vi "Stop Core.vi"(10 "final error code":i32, 11 "CS++RTRootActor in":refnum<class "CS++RTRootActor.lvclass">) -> (3 "CS++RTRootActor out":refnum<class "CS++RTRootActor.lvclass">)   [LabVIEW 2014, in "CS++RTRoot.lvlib" / "CS++RTRootActor.lvclass"]
doc: "(<B>Filename</B>: Actor Framework.lvlib:Actor.lvclass:Stop Core.vi)\n\nDefines what the actor does before it stops. Use the <B>final error code</B> input to determine whether the actor shut down in response to an error.\n\nBy default, this method does nothing. A descendant class may override it to define behavior, such as shutting down any processes the actor initiated in its override of the Actor Core method."
uses:
  CS++RTRootActor.lvclass
  <vilib>/ActorFramework/Actor/Actor.lvclass
  CSPP_Core/Libraries/Utilities/CS++Utilities.lvlib
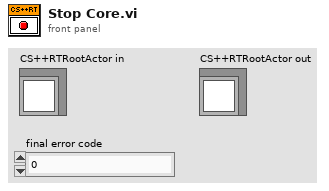
[diagram p1: front panel]
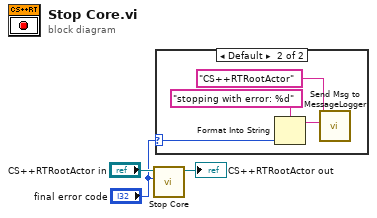
[diagram p0: block diagram]
diagram:
  n1 = call-parent "Stop Core.vi"("final error code"="final error code", "Actor in"="CS++RTRootActor in") -> ("Actor out"=→"CS++RTRootActor out":refnum<class "CS++RTRootActor.lvclass">)  [unwired: 9 in]
  n2 = case shown="Default" "final error code" {
    selector: "final error code" -> [_ w6]
    frame 0 {
    }
    frame Default {
      n3 = Format Into String(format string="stopping with error: %d", w6) -> (resulting string=w4:string)  [unwired: 2 in, 1 out]
      n4 = call "Send Msg to MessageLogger.vi"("Message Content"=w4, "Message Tag"="CS++RTRootActor" ("String to write")) -> ()  [unwired: 9 in, 1 out]
    }
  }
